vi "sub_joystick_to_SRC-cmd.vi"(8 "error in":errorcluster, 11 "index":u8) -> (0 "error out":errorcluster, 3 "cmd out":string)   [LabVIEW 2019]
uses:
  Ctrl/cmd_common.ctl
  Ctrl/joystick_opval.ctl
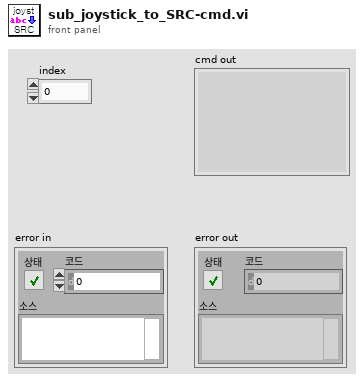
[diagram p1: front panel]
types:
  T1 = typedef "cmd_common.ctl" = enum16{"read", "write"}
  T2 = typedef "joystick_opval.ctl" = cluster{"curr":u32, "last":u32}
  T3 = typedef "joystick cfg.ctl" = cluster{"Type":enum16{"Logitech F710", "Xbox"}, "steer limit":cluster{"min":dbl, "max":dbl, "scale":dbl, "offset":dbl}, "speed limit":cluster{"min":dbl, "max":dbl, "pwm max":dbl}, "ID":i32, "joystick max":dbl}
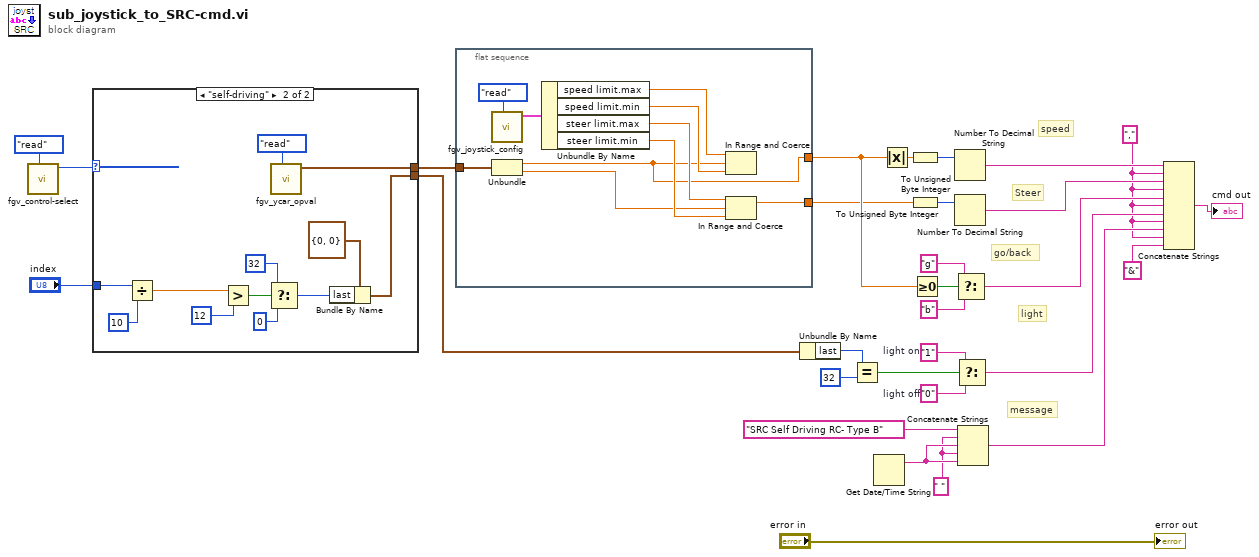
[diagram p0: block diagram]
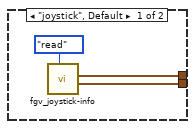
[diagram p2: hidden frame]
diagram:
  w20 = "0"  # light off
  w19 = "1"  # light on
  w17 = " " ("문자열")
  w14 = "," ("string")
  # "message"
  # "light"
  # "go/back"
  # "Steer"
  # "speed"
  n1 = call "fgv_control-select.vi"("cmd"=cmd_common."read") -> ("mode out"=w6:enum16{"joystick", "self-driving"})  [unwired: 10 in]
  n2 = case shown="\"self-driving\"" w6 {
    tunnel: [w33 w42] -> w3
    tunnel: [w32 w44] -> w4
    tunnel: "index" -> [_ w36]
    frame "joystick", Default {
      n3 = call "fgv_joystick-info.vi"("init"=enum16{"enable", "init", "read", "write"}."read") -> ("opval"=w33:T2, "v_val"=w32:cluster{dbl, dbl})  [unwired: 7 in, 2 out]
    }
    frame "self-driving" {
      n4 = Divide(x=w36, y=u8 10) -> (x/y=w34:dbl)
      n5 = Greater?(x=w34, y=u8 12) -> (0:w40:bool)
      n6 = Select(t=u8 32 ("y"), s=w40, f=u8 0 ("y")) -> (s? t:f=w41:u8)
      n7 = call "fgv_ycar_opval.vi"("cmd"=enum16{"read", "write", "ini"}."read") -> ("opval out"=w44:cluster{"speed":dbl, "steer":dbl})  [unwired: 10 in]
      n8 = Bundle By Name(cluster=T2 {"curr"=0, "last"=0} ("opval"), "last"=w41) -> (w42:T2)
    }
  }
  n9 = flat-sequence {
    tunnel: w4 -> [w54]
    tunnel: [w46] -> w2
    tunnel: [w47] -> w1
    frame #0 {
      n10 = call "fgv_joystick_config.vi"("cmd"=cmd_common."read") -> ("Joystick cfg out"=w53:T3)  [unwired: 9 in, 1 out]
      n11 = Unbundle(w54) -> ("speed"=w46:dbl, "steer"=w48:dbl)
      n12 = Unbundle By Name(w53) -> ("speed limit.max"=w52:dbl, "speed limit.min"=w51:dbl, "steer limit.max"=w50:dbl, "steer limit.min"=w49:dbl)
      n13 = In Range and Coerce(upper limit=w52, x=w46, lower limit=w51) -> ()  [unwired: 2 out]
      n14 = In Range and Coerce(upper limit=w50, x=w48, lower limit=w49) -> (coerced(x)=w47:dbl)  [unwired: 1 out]
    }
  }
  n15 = Unbundle By Name(w3) -> ("last"=w28:u32)
  n16 = Equal?(x=w28, y=u32 32) -> (x = y?=w29:bool)
  n17 = Get Date/Time String() -> (date string=w26:string)  [unwired: 3 in, 1 out]
  n18 = Absolute Value(x=w2) -> (abs(x)=w9:dbl)
  n19 = To Unsigned Byte Integer(number=w9) -> (unsigned 8bit integer=w7:u8)
  n20 = To Unsigned Byte Integer(number=w1) -> (unsigned 8bit integer=w8:u8)
  n21 = Greater Or Equal To 0?(x=w2) -> (x >= 0?=w24:bool)
  n22 = Number To Decimal String(number=w7) -> (decimal integer string=w22:string)  [unwired: 1 in]
  n23 = Number To Decimal String(number=w8) -> (decimal integer string=w23:string)  [unwired: 1 in]
  n24 = Select(t="g" ("string"), s=w24, f="b" ("string")) -> (s? t:f=w25:string)
  n25 = Select(t=w19, s=w29, f=w20) -> (s? t:f=w27:string)
  n26 = Concatenate Strings("SRC Self Driving RC- Type B" ("문자열"), w17, w26, w17, w26) -> (w30:string)
  n27 = Concatenate Strings(w22, w14, w23, w14, w25, w14, w27, w14, w30, w14, "&" ("string")) -> (→"cmd out":string)
  "error out" <- "error in"
